vi "ColorDetection23.vi"() -> ()   [LabVIEW 2018]
uses:
  Control 1.ctl
  <vilib>/myRIO/Instrument Drivers/Onboard IO/DIO/typedefs/DIO Reference.ctl
  <vilib>/myRIO/Common/Instrument Driver Framework/Utilities/typedefs/myRIO Generic Hardware Reference.ctl
  <vilib>/myRIO/Common/Instrument Driver Framework/Utilities/typedefs/Hardware Version Enum.ctl
  <vilib>/myRIO/Common/Instrument Driver Framework/Utilities/typedefs/myRIO v1.0 Reference.ctl
  <vilib>/myRIO/Common/Instrument Driver Framework/Utilities/typedefs/Generic FPGA Reference.ctl
  <vilib>/myRIO/Common/Instrument Driver Framework/myRIO v1.0/DIO/typedefs/DIO Channels List.ctl
  <vilib>/myRIO/Common/Instrument Driver Framework/myRIO v1.0/DIO/typedefs/DIO Channels Enum.ctl
  <vilib>/userdefined/High Color/nirio_resource_hc.ctl
  <vilib>/myRIO/Common/Instrument Driver Framework/Utilities/vis/Is FPGA Ref Available.vi
  <vilib>/myRIO/Common/Instrument Driver Framework/myRIO v1.0/DIO/vis/myRIO v1.1 Open DIO.vi
  <vilib>/myRIO/Instrument Drivers/Onboard IO/DIO/vis/Write.vi
  <vilib>/myRIO/Common/Instrument Driver Framework/Utilities/vis/Validate Channels.vi
  <vilib>/myRIO/Common/Instrument Driver Framework/myRIO v1.0/DIO/vis/myRIO v1.0 Reserve DIO.vi
  <vilib>/myRIO/Common/Instrument Driver Framework/myRIO v1.0/UART/vis/myRIO v1.0 Close UART.vi
  <vilib>/myRIO/Common/Instrument Driver Framework/myRIO v1.0/Resource Manager/vis/myRIO v1.0 Reserve Channel List.vi
  <vilib>/myRIO/Common/Instrument Driver Framework/myRIO v1.0/DIO/vis/myRIO v1.0 Build MUX Configuration DIO.vi
  <vilib>/myRIO/Common/Instrument Driver Framework/myRIO v1.0/Resource Manager/vis/myRIO v1.0 Reserve Channel.vi
  <vilib>/myRIO/Common/Instrument Driver Framework/myRIO v1.0/Resource Manager/vis/myRIO v1.0 Unreserve Channel.vi
  <vilib>/myRIO/Common/Instrument Driver Framework/myRIO v1.0/Resource Manager/vis/myRIO v1.0 Create Configuration List.vi
  <vilib>/myRIO/Common/Instrument Driver Framework/myRIO v1.0/Resource Manager/vis/myRIO v1.0 Build Mutex Name.vi
  <vilib>/Utility/VariantDataType/GetNumericInfo.vi
  <vilib>/Utility/error.llb/Error Cluster From Error Code.vi
  <vilib>/myRIO/Common/Instrument Driver Framework/myRIO v1.0/myRIO v1.1 Open.vi
  <vilib>/myRIO/Common/Instrument Driver Framework/Utilities/vis/IO Manager.vi
  <vilib>/myRIO/Common/Instrument Driver Framework/Utilities/vis/Configuration Manager.vi
  <vilib>/myRIO/Common/Instrument Driver Framework/myRIO v1.0/Resource Manager/vis/myRIO v1.0 Configure IO.vi
  <vilib>/myRIO/Common/Instrument Driver Framework/myRIO v1.0/myRIO v1.0 Close.vi
  <vilib>/myRIO/Common/Instrument Driver Framework/myRIO v1.0/DIO/vis/myRIO v1.0 Write DIO.vi
  <vilib>/myRIO/Common/Instrument Driver Framework/Utilities/vis/FPGA Ref Manager.vi
  <vilib>/myRIO/Common/Instrument Driver Framework/myRIO v1.0/myRIO v1.0 Reset FPGA.vi
  <vilib>/myRIO/Common/Instrument Driver Framework/myRIO v1.0/IRQ/vis/myRIO v1.0 IRQ Info FGV.vi
  <vilib>/myRIO/Common/Instrument Driver Framework/myRIO v1.0/IRQ/vis/myRIO v1.0 Timer IRQ Info FGV.vi
  <vilib>/myRIO/Common/Instrument Driver Framework/myRIO v1.0/IRQ/vis/myRIO v1.0 ISR Agent.vi
  <vilib>/myRIO/Express VI/Onboard IO/DO/DO Express VI.xnode
  <vilib>/myRIO/Instrument Drivers/Onboard IO/DIO/vis/myRIO DIO Open.xnode
  <vilib>/myRIO/Instrument Drivers/Utilities/Utilities.lvlib
  <vilib>/vision/NI_Vision_Development_Module.lvlib
  <vilib>/myRIO/Instrument Drivers/Onboard IO/DIO/DIO.lvlib
panel:
  out "Negro":bool
  out "Amarillo":bool
  out "Rojo":bool
  out "Azul":bool
  out "Verde":bool
  out "Enum":T1
  out "Color Spectrum 3":dbl[](array[numeric]) format="%.2f"
  out "Color Spectrum 2":dbl[](array[numeric]) format="%.2f"
  out "Azul  3":bool
  out "Negro 3":bool
  out "Amarillo 3":bool
  out "Verde 3":bool
  out "Rojo 3":bool
  out "Azul  2":bool
  out "Negro 2":bool
  out "Amarillo 2":bool
  out "Verde 2":bool
  out "Rojo 2":bool
  out "Banda 1 H1":bool
  out "Banda 1 H0":bool
  out "Image Out":T2(plugin-control)
  in  "Stop (F)":bool
  out "Color Spectrum":dbl[](array[numeric]) format="%.2f"
  # "Seccion 1"
  # "Seccion 2"
  # "Seccion 3"
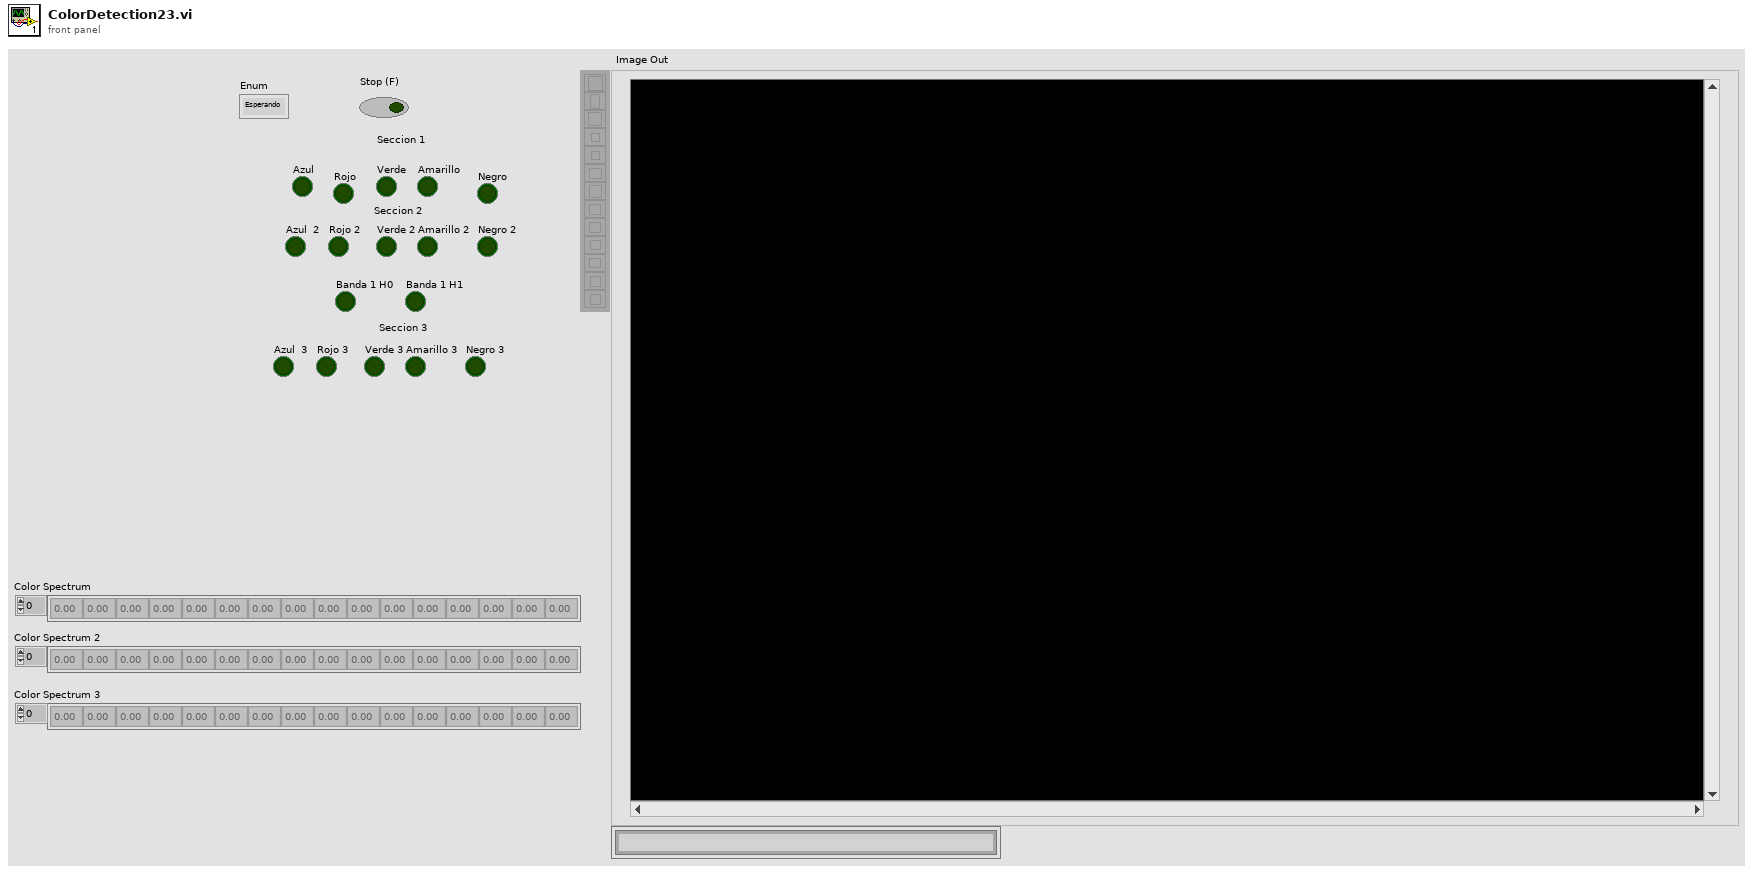
[diagram p1: front panel]
types:
  T1 = typedef "Control 1.ctl" = enum16{"Esperando", "Seccion1", "Seccion2", "Seccion3", "Seccion4", "Seccion5", "Seccion6", "Seccion7"}
  T2 = typedef "IMAQ Image.ctl" = refnum<image>
  T3 = typedef "IMAQ Rectangle" = cluster{"Left":i32, "Top":i32, "Right":i32, "Bottom":i32, "Rotation":dbl}
  T4 = typedef "DIO.lvlib/DIO Reference.ctl" = cluster{"myRIO Reference":T5, "DIO Channels List":T9}
  T5 = typedef "myRIO Generic Hardware Reference.ctl" = cluster{"myRIO Model":T6, "myRIO Hardware Reference":T7}
  T6 = typedef "Hardware Version Enum.ctl" = enum16{"Unknown", "myRIO-1900", "myRIO-1950", "roboRIO", "NI ELVIS RIO CM", "ELVIS III"}
  T7 = typedef "myRIO v1.0 Reference.ctl" = cluster{"Generic FPGA Reference":T8, "Allow multiple opens":bool}
  T8 = typedef "Generic FPGA Reference.ctl" = refnum<k20>
  T9 = typedef "DIO Channels List.ctl" = T10[]
  T10 = typedef "DIO Channels Enum.ctl" = enum16{"Not Connected", "C/DIO0", "C/DIO1", "C/DIO2", "C/DIO3", "C/DIO4", "C/DIO5", "C/DIO6", "C/DIO7", "A/DIO0", "A/DIO1", "A/DIO2", "A/DIO3", "A/DIO4", "A/DIO5", "A/DIO6", "A/DIO7", "A/DIO8", "A/DIO9", "A/DIO10", "A/DIO11", "A/DIO12", "A/DIO13", "A/DIO14", "A/DIO15", "A/DIO16", "A/DIO17", "A/DIO18", "A/DIO19", "B/DIO0", "B/DIO1", "B/DIO2", "B/DIO3", "B/DIO4", "B/DIO5", "B/DIO6", "B/DIO7", "B/DIO8", "B/DIO9", "B/DIO10", "B/DIO11", "B/DIO12", "B/DIO13", "B/DIO14", "B/DIO15", "B/DIO16", "B/DIO17", "B/DIO18", "B/DIO19", "LED0", "LED1", "LED2", "LED3", "Button0", "DIO/DIO0", "DIO/DIO1", "DIO/DIO2", "DIO/DIO3", "DIO/DIO4", "DIO/DIO5", "DIO/DIO6", "DIO/DIO7", "DIO/DIO8", "DIO/DIO9", "SPI/CS0", "SPI/CS1", "SPI/CS2", "SPI/CS3", "LED RADIO (Green)", "LED RADIO (Red)", "LED COMM (Green)", "LED COMM (Red)", "LED MODE (Green)", "LED MODE (Red)"}
  T11 = typedef "nirio_resource_hc.ctl" = tag
  T12 = typedef "ROI Descriptor" = cluster{"Global Rectangle":i32[], "Contours":cluster{"ID":enum32{"External", "Internal"}, "Type":u32, "Coordinates":i32[]}[]}
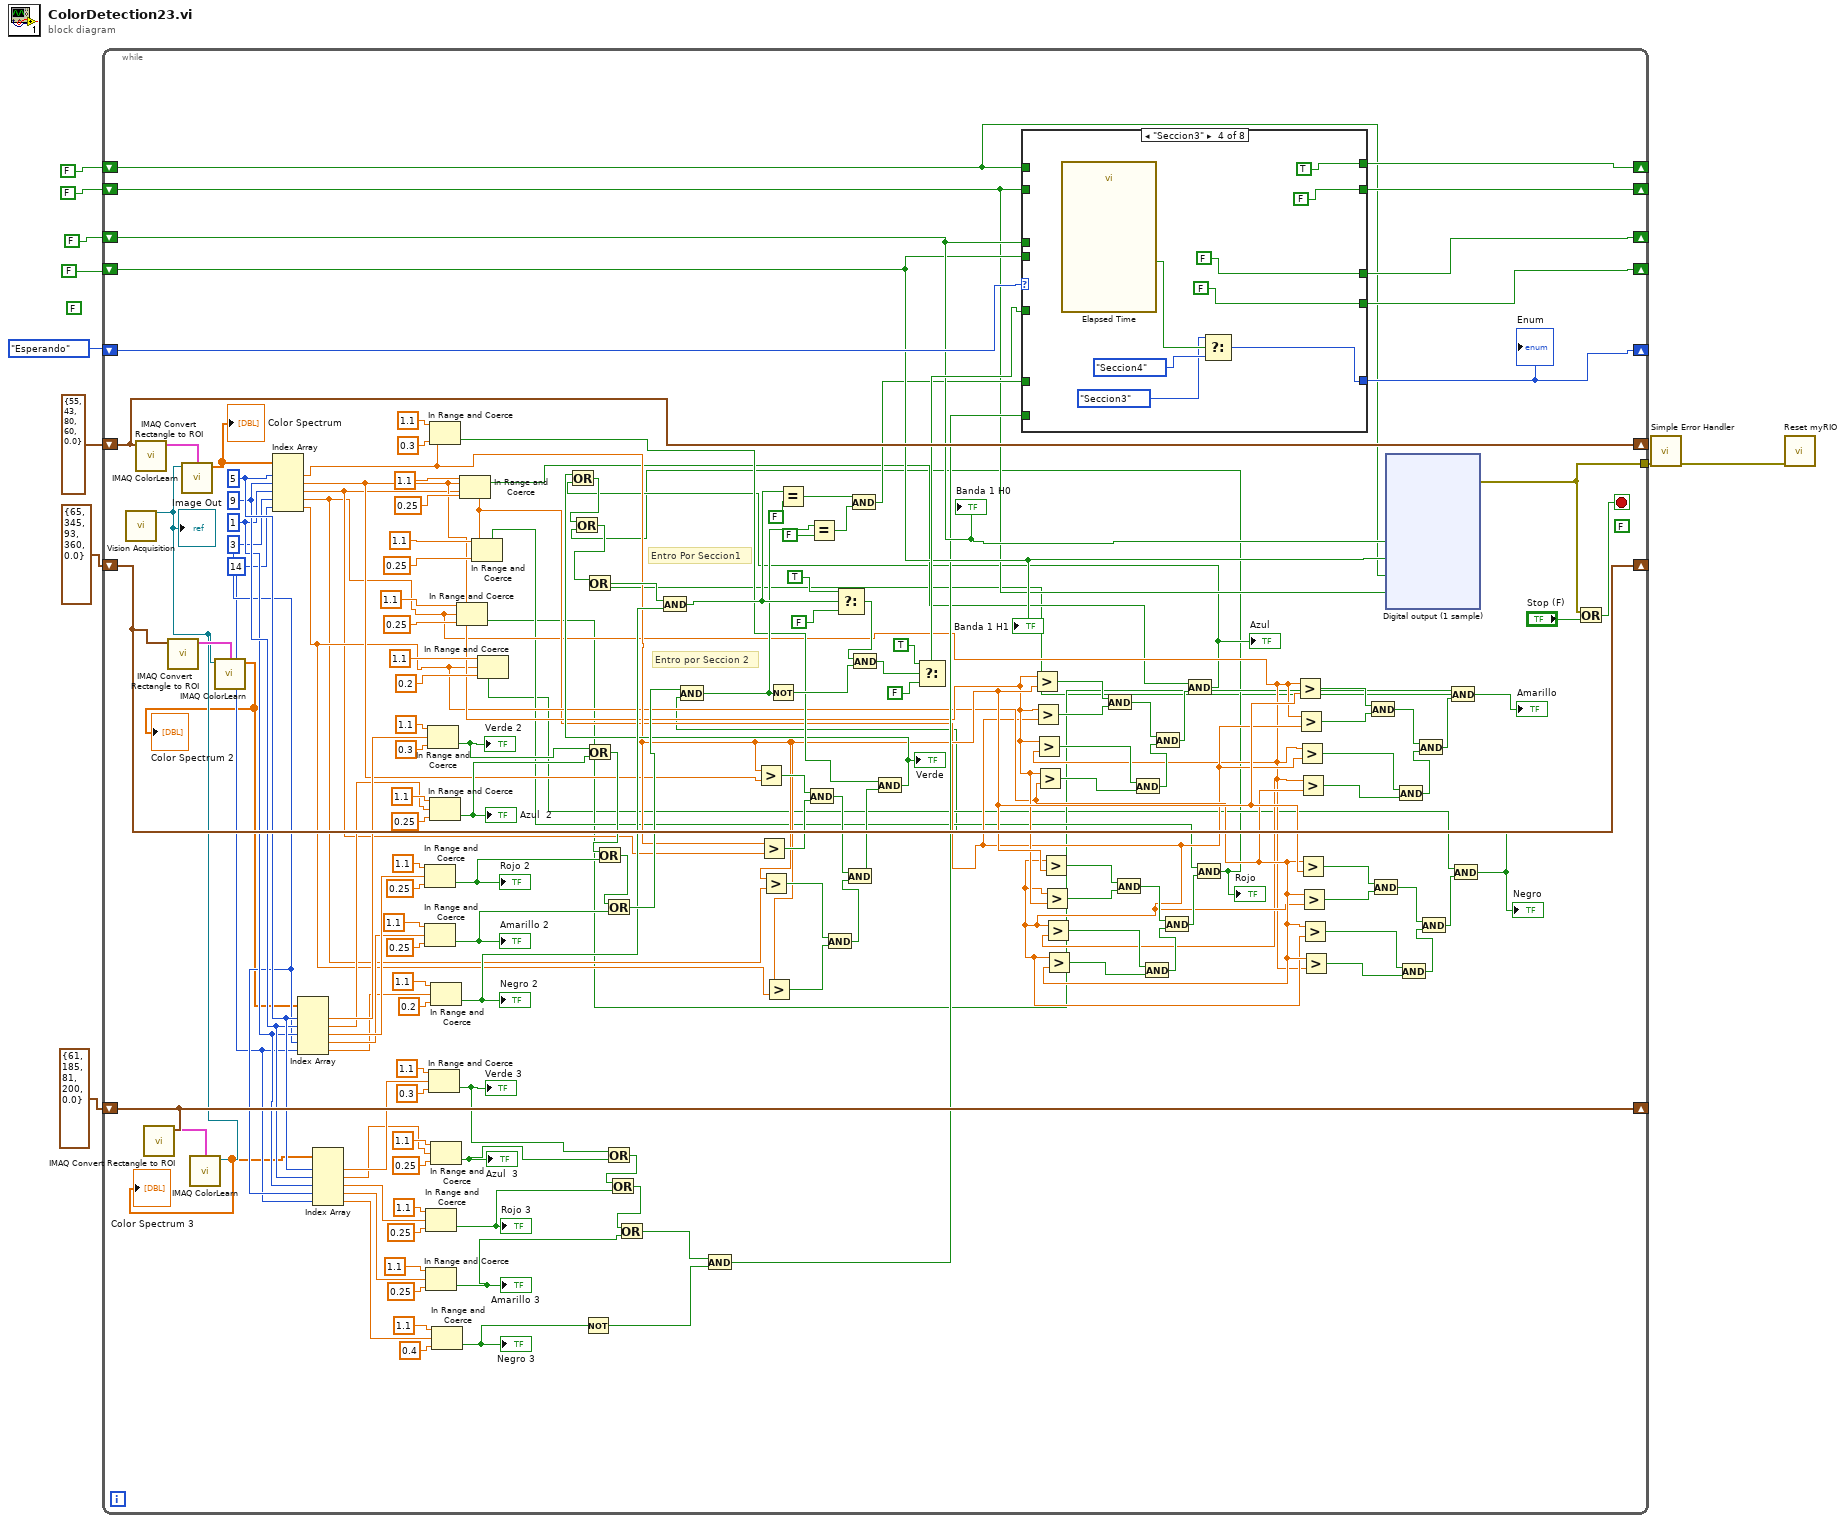
[diagram p0: block diagram]
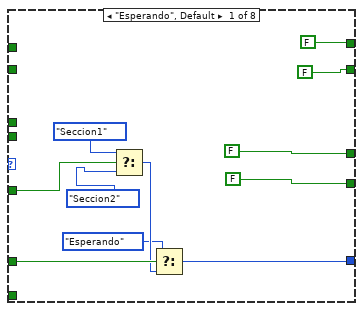
[diagram p2: hidden frame]
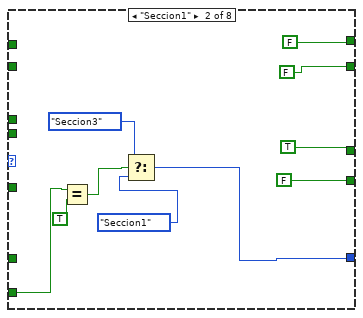
[diagram p3: hidden frame]
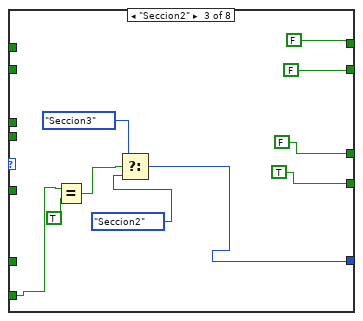
[diagram p4: hidden frame]
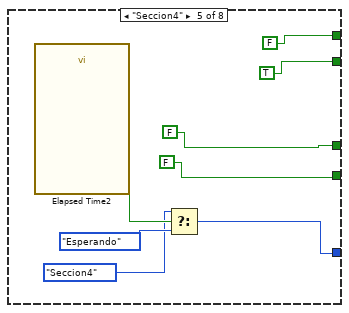
[diagram p5: hidden frame]
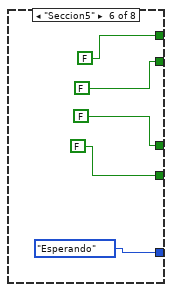
[diagram p6: hidden frame]
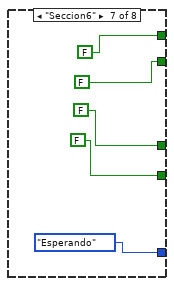
[diagram p7: hidden frame]
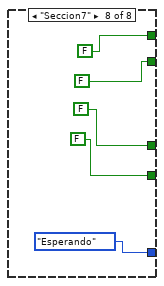
[diagram p8: hidden frame]
diagram:
  (unwired) FALSE
  n1 = while {
    shift-right: [w156] -> _
    shift-left: T3 {"Left"=55, "Top"=43, "Right"=80, "Bottom"=60, "Rotation"=0.0} ("Rectangle") -> [w156]
    tunnel: [w150] -> w8
    shift-right: [w148] -> _
    shift-left: T3 {"Left"=65, "Top"=345, "Right"=93, "Bottom"=360, "Rotation"=0.0} ("Rectangle") -> [w148]
    shift-right: [w121] -> _
    shift-left: T3 {"Left"=61, "Top"=185, "Right"=81, "Bottom"=200, "Rotation"=0.0} ("Rectangle") -> [w121]
    shift-right: [w85] -> _
    shift-left: FALSE -> [w74]
    shift-right: [w84] -> _
    shift-left: FALSE -> [w73]
    shift-right: [w83] -> _
    shift-left: Control_1."Esperando" -> [w86]
    shift-right: [w64] -> _
    shift-left: FALSE -> [w62]
    shift-right: [w63] -> _
    shift-left: FALSE -> [w61]
    stop <- w149 stop-if-true
    (unwired) FALSE
    w115 = 3 ("index")
    w114 = 14 ("index")
    w116 = 1 ("index")
    w117 = 9 ("index")
    w118 = 5 ("index")
    # "Entro por Seccion 2"
    # "Entro Por Seccion1"
    n2 = call "Vision Acquisition"() -> ("Image Out"=w120:T2)  [unwired: 25 in, 2 out]
    "Image Out" <- w120
    n3 = call "IMAQ Convert Rectangle to ROI"("Rectangle"=w156) -> ("ROI Descriptor"=w153:T12)  [unwired: 8 in, 1 out]
    n4 = call "IMAQ Convert Rectangle to ROI"("Rectangle"=w121) -> ("ROI Descriptor"=w119:T12)  [unwired: 8 in, 1 out]
    n5 = call "IMAQ Convert Rectangle to ROI"("Rectangle"=w148) -> ("ROI Descriptor"=w147:T12)  [unwired: 8 in, 1 out]
    n6 = call "IMAQ ColorLearn"("ROI Descriptor"=w153, "Image"=w120) -> ("Color Spectrum"=w152:dbl[])  [unwired: 6 in, 1 out]
    "Color Spectrum" <- w152
    n7 = call "IMAQ ColorLearn"("ROI Descriptor"=w119, "Image"=w120) -> ("Color Spectrum"=w98:dbl[])  [unwired: 6 in, 1 out]
    "Color Spectrum 3" <- w98
    n8 = call "IMAQ ColorLearn"("ROI Descriptor"=w147, "Image"=w120) -> ("Color Spectrum"=w97:dbl[])  [unwired: 6 in, 1 out]
    "Color Spectrum 2" <- w97
    n9 = Index Array(array=w152, index #1=w118, index #2=w117, index #3=w116, index #4=w115, index #5=w114) -> (element #1=w23:dbl, element #2=w22:dbl, element #3=w20:dbl, element #4=w19:dbl, element #5=w21:dbl)
    n10 = Index Array(array=w97, index #1=w118, index #2=w117, index #3=w116, index #4=w115, index #5=w114) -> (element #1=w136:dbl, element #2=w135:dbl, element #3=w134:dbl, element #4=w133:dbl, element #5=w132:dbl)
    n11 = Index Array(array=w98, index #1=w118, index #2=w117, index #3=w116, index #4=w115, index #5=w114) -> (element #1=w103:dbl, element #2=w102:dbl, element #3=w101:dbl, element #4=w100:dbl, element #5=w99:dbl)
    n12 = In Range and Coerce(upper limit=1.1, x=w134, lower limit=0.25) -> (In Range?=w127:bool)  [unwired: 1 out]
    "Rojo 2" <- w127
    n13 = In Range and Coerce(upper limit=1.1, x=w133, lower limit=0.25) -> (In Range?=w126:bool)  [unwired: 1 out]
    "Amarillo 2" <- w126
    n14 = In Range and Coerce(upper limit=1.1, x=w101, lower limit=0.25) -> (In Range?=w93:bool)  [unwired: 1 out]
    "Rojo 3" <- w93
    n15 = In Range and Coerce(upper limit=1.1, x=w100, lower limit=0.25) -> (In Range?=w91:bool)  [unwired: 1 out]
    "Amarillo 3" <- w91
    n16 = In Range and Coerce(upper limit=1.1, x=w136, lower limit=0.3) -> (In Range?=w129:bool)  [unwired: 1 out]
    "Verde 2" <- w129
    n17 = In Range and Coerce(upper limit=1.1, x=w103, lower limit=0.3) -> (In Range?=w96:bool)  [unwired: 1 out]
    "Verde 3" <- w96
    n18 = In Range and Coerce(upper limit=1.1, x=w23, lower limit=0.3) -> (In Range?=w53:bool)  [unwired: 1 out]
    n19 = In Range and Coerce(upper limit=1.1, x=w135, lower limit=0.25) -> (In Range?=w128:bool)  [unwired: 1 out]
    "Azul  2" <- w128
    n20 = In Range and Coerce(upper limit=1.1, x=w132, lower limit=0.2) -> (In Range?=w87:bool)  [unwired: 1 out]
    "Negro 2" <- w87
    n21 = In Range and Coerce(upper limit=1.1, x=w102, lower limit=0.25) -> (In Range?=w95:bool)  [unwired: 1 out]
    "Azul  3" <- w95
    n22 = In Range and Coerce(upper limit=1.1, x=w99, lower limit=0.4) -> (In Range?=w90:bool)  [unwired: 1 out]
    "Negro 3" <- w90
    n23 = In Range and Coerce(upper limit=1.1, x=w19, lower limit=0.25) -> (In Range?=w16:bool)  [unwired: 1 out]
    n24 = In Range and Coerce(upper limit=1.1, x=w22, lower limit=0.25) -> (In Range?=w18:bool)  [unwired: 1 out]
    n25 = In Range and Coerce(upper limit=1.1, x=w20, lower limit=0.25) -> (In Range?=w17:bool)  [unwired: 1 out]
    n26 = In Range and Coerce(upper limit=1.1, x=w21, lower limit=0.2) -> (In Range?=w15:bool)  [unwired: 1 out]
    n27 = Not(x=w90) -> (.not. x?=w89:bool)
    n28 = Or(x=w129, y=w128) -> (x .or. y?=w124:bool)
    n29 = Or(x=w124, y=w127) -> (x .or. y?=w125:bool)
    n30 = Or(x=w125, y=w126) -> (x .or. y?=w122:bool)
    n31 = Or(x=w96, y=w95) -> (x .or. y?=w94:bool)
    n32 = Or(x=w94, y=w93) -> (x .or. y?=w92:bool)
    n33 = Or(x=w92, y=w91) -> (x .or. y?=w88:bool)
    n34 = And(x=w88, y=w89) -> (x .and. y?=w65:bool)
    n35 = Greater?(x=w23, y=w22) -> (0:w60:bool)
    n36 = Greater?(x=w23, y=w20) -> (0:w59:bool)
    n37 = Greater?(x=w23, y=w19) -> (0:w58:bool)
    n38 = Greater?(x=w23, y=w21) -> (0:w57:bool)
    n39 = And(x=w60, y=w59) -> (x .and. y?=w56:bool)
    n40 = And(x=w58, y=w57) -> (x .and. y?=w55:bool)
    n41 = And(x=w56, y=w55) -> (x .and. y?=w54:bool)
    n42 = And(x=w53, y=w54) -> (x .and. y?=w52:bool)
    "Verde" <- w52
    n43 = Greater?(x=w22, y=w23) -> (0:w51:bool)
    n44 = Greater?(x=w22, y=w20) -> (0:w50:bool)
    n45 = Greater?(x=w22, y=w19) -> (0:w49:bool)
    n46 = Greater?(x=w22, y=w21) -> (0:w48:bool)
    n47 = Greater?(x=w20, y=w23) -> (0:w44:bool)
    n48 = Greater?(x=w20, y=w22) -> (0:w43:bool)
    n49 = Greater?(x=w20, y=w19) -> (0:w42:bool)
    n50 = Greater?(x=w20, y=w21) -> (0:w41:bool)
    n51 = And(x=w51, y=w50) -> (x .and. y?=w46:bool)
    n52 = And(x=w44, y=w43) -> (x .and. y?=w39:bool)
    n53 = And(x=w49, y=w48) -> (x .and. y?=w47:bool)
    n54 = And(x=w42, y=w41) -> (x .and. y?=w40:bool)
    n55 = And(x=w46, y=w47) -> (x .and. y?=w45:bool)
    n56 = And(x=w39, y=w40) -> (x .and. y?=w38:bool)
    n57 = And(x=w18, y=w45) -> (x .and. y?=w14:bool)
    "Azul" <- w14
    n58 = Or(x=w52, y=w14) -> (x .or. y?=w131:bool)
    n59 = And(x=w17, y=w38) -> (x .and. y?=w13:bool)
    "Rojo" <- w13
    n60 = Or(x=w131, y=w13) -> (x .or. y?=w130:bool)
    n61 = Greater?(x=w19, y=w23) -> (0:w37:bool)
    n62 = Greater?(x=w19, y=w20) -> (0:w36:bool)
    n63 = Greater?(x=w19, y=w20) -> (0:w35:bool)
    n64 = Greater?(x=w19, y=w21) -> (0:w34:bool)
    n65 = Greater?(x=w21, y=w23) -> (0:w30:bool)
    n66 = Greater?(x=w21, y=w20) -> (0:w29:bool)
    n67 = Greater?(x=w21, y=w20) -> (0:w28:bool)
    n68 = Greater?(x=w21, y=w19) -> (0:w27:bool)
    n69 = And(x=w37, y=w36) -> (x .and. y?=w32:bool)
    n70 = And(x=w30, y=w29) -> (x .and. y?=w25:bool)
    n71 = xnode "Digital output (1 sample)"("h0 (B/DIO1 (Pin 13))"=w74, "h1 (B/DIO0 (Pin 11))"=w73, "h2 (B/DIO2 (Pin 15))"=w62, "h3 (B/DIO3 (Pin 17))"=w61) -> ("error out"=w150:errorcluster)  [unwired: 1 in]
    n72 = And(x=w35, y=w34) -> (x .and. y?=w33:bool)
    n73 = And(x=w28, y=w27) -> (x .and. y?=w26:bool)
    n74 = And(x=w32, y=w33) -> (x .and. y?=w31:bool)
    n75 = And(x=w25, y=w26) -> (x .and. y?=w24:bool)
    n76 = And(x=w16, y=w31) -> (x .and. y?=w12:bool)
    "Amarillo" <- w12
    n77 = Or(x=w130, y=w12) -> (x .or. y?=w123:bool)
    n78 = And(x=w123, y=w87) -> (x .and. y?=w72:bool)
    n79 = Equal?(x=w72, y=FALSE) -> (x = y?=w68:bool)
    n80 = Select(t=TRUE, s=w72, f=FALSE) -> (s? t:f=w79:bool)
    n81 = And(x=w15, y=w24) -> (x .and. y?=w11:bool)
    "Negro" <- w11
    n82 = And(x=w122, y=w11) -> (x .and. y?=w70:bool)
    n83 = Not(x=w70) -> (.not. x?=w78:bool)
    n84 = Equal?(x=w70, y=FALSE) -> (x = y?=w67:bool)
    n85 = And(x=w68, y=w67) -> (x .and. y?=w66:bool)
    n86 = And(x=w79, y=w78) -> (x .and. y?=w77:bool)
    n87 = Select(t=TRUE, s=w77, f=FALSE) -> (s? t:f=w80:bool)
    n88 = case shown="\"Seccion3\"" w86 {
      tunnel: [FALSE TRUE ("y") FALSE FALSE FALSE FALSE FALSE FALSE] -> w85
      tunnel: [FALSE FALSE ("y") TRUE FALSE FALSE FALSE FALSE FALSE] -> w84
      tunnel: [w167 w178 w188 w198 w206 Control_1."Esperando" Control_1."Esperando" Control_1."Esperando"] -> w83
      tunnel: w80 -> [w173 _ _ _ _ _ _ _]
      tunnel: w74 -> [_ _ _ _ _ _ _ _]
      tunnel: w73 -> [_ _ _ _ _ _ _ _]
      tunnel: w66 -> [w170 _ _ _ _ _ _ _]
      tunnel: w65 -> [_ w185 w189 _ _ _ _ _]
      tunnel: w61 -> [_ _ _ _ _ _ _ _]
      tunnel: w62 -> [_ _ _ _ _ _ _ _]
      tunnel: [FALSE FALSE FALSE TRUE FALSE FALSE FALSE FALSE] -> w64
      tunnel: [FALSE FALSE FALSE FALSE TRUE FALSE FALSE FALSE] -> w63
      frame "Esperando", Default {
        n89 = Select(t=Control_1."Seccion1", s=w173, f=Control_1."Seccion2") -> (s? t:f=w169:T1)
        n90 = Select(t=Control_1."Esperando", s=w170, f=w169) -> (s? t:f=w167:T1)
      }
      frame "Seccion1" {
        n91 = Equal?(x=w185, y=TRUE) -> (x = y?=w183:bool)
        n92 = Select(t=Control_1."Seccion3", s=w183, f=Control_1."Seccion1") -> (s? t:f=w178:T1)
      }
      frame "Seccion2" {
        n93 = Equal?(x=w189, y=TRUE) -> (x = y?=w192:bool)
        n94 = Select(t=Control_1."Seccion3", s=w192, f=Control_1."Seccion2") -> (s? t:f=w188:T1)
      }
      frame "Seccion3" {
        n95 = call "Elapsed Time"() -> ("Time has Elapsed"=w201:bool)  [unwired: 12 in, 7 out]
        n96 = Select(t=Control_1."Seccion3", s=w201, f=Control_1."Seccion4") -> (s? t:f=w198:T1)
      }
      frame "Seccion4" {
        n97 = call "Elapsed Time2"() -> ("Time has Elapsed"=w211:bool)  [unwired: 12 in, 7 out]
        n98 = Select(t=Control_1."Seccion4", s=w211, f=Control_1."Esperando") -> (s? t:f=w206:T1)
      }
      frame "Seccion5" {
      }
      frame "Seccion6" {
      }
      frame "Seccion7" {
      }
    }
    "Enum" <- w83
    n99 = Or(x=w150, y="Stop (F)") -> (x .or. y?=w149:bool)
    "Banda 1 H0" <- w74
    "Banda 1 H1" <- w73
  }
  n100 = call <vilib>:"Simple Error Handler.vi"("error in (no error)"=w8) -> ("error out"=w9:errorcluster)  [unwired: 4 in, 4 out]
  n101 = call <vilib>:"Reset myRIO.vi"("error in (no error)"=w9) -> ()  [unwired: 10 in, 1 out]
